vi "SetAnalogOutUI.vi"(8 "Error in":errorcluster, 11 "DevicesAndSignals":T1) -> (0 "Error out":errorcluster, 3 "DevicesAndSignals":T1)   [LabVIEW 2016]
doc: "Use this VI to set selected analog out signals to a certain value."
panel:
  in  "?":dbl(slide) min=-10.0 max=10.0 step=0.01 scale=-10.0..10.0 scale format="%.1g"
  in  "SetAnalogOut":bool
  in  "Signals":i32(listbox)
  in  "stop":bool caption="Stopp"
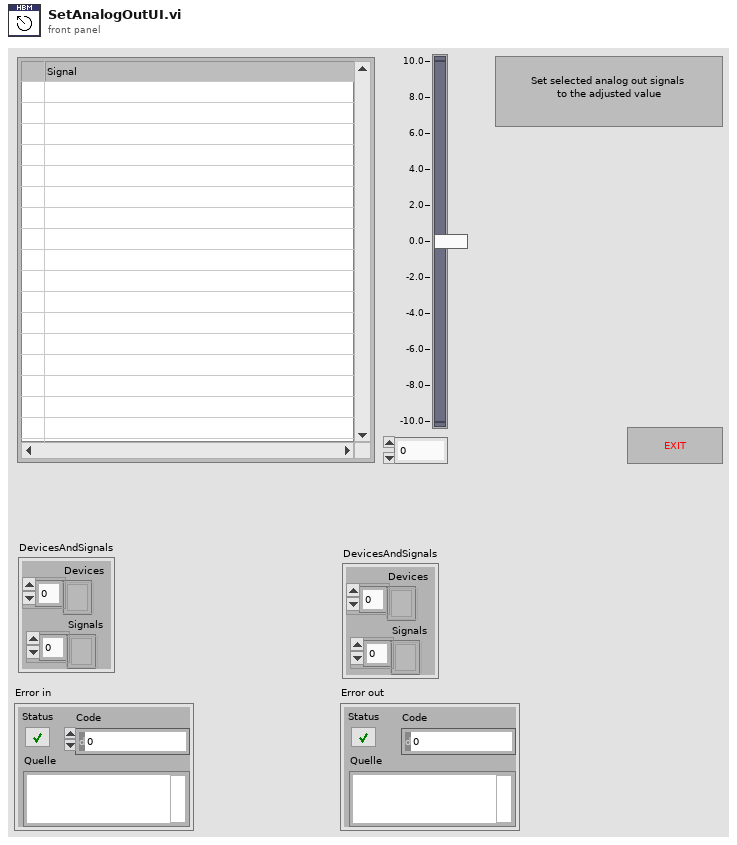
[diagram p1: front panel]
types:
  T1 = cluster{"Devices":refnum<k24>[], "Signals":refnum<k24>[]}
  T2 = typedef "LVPoint32TypeDef.ctl" = cluster{"Horizontal":i32, "Vertical":i32}
  T3 = typedef "LVRowAndColumnTypeDef.ctl" = cluster{"Row":i32, "Column":i32}
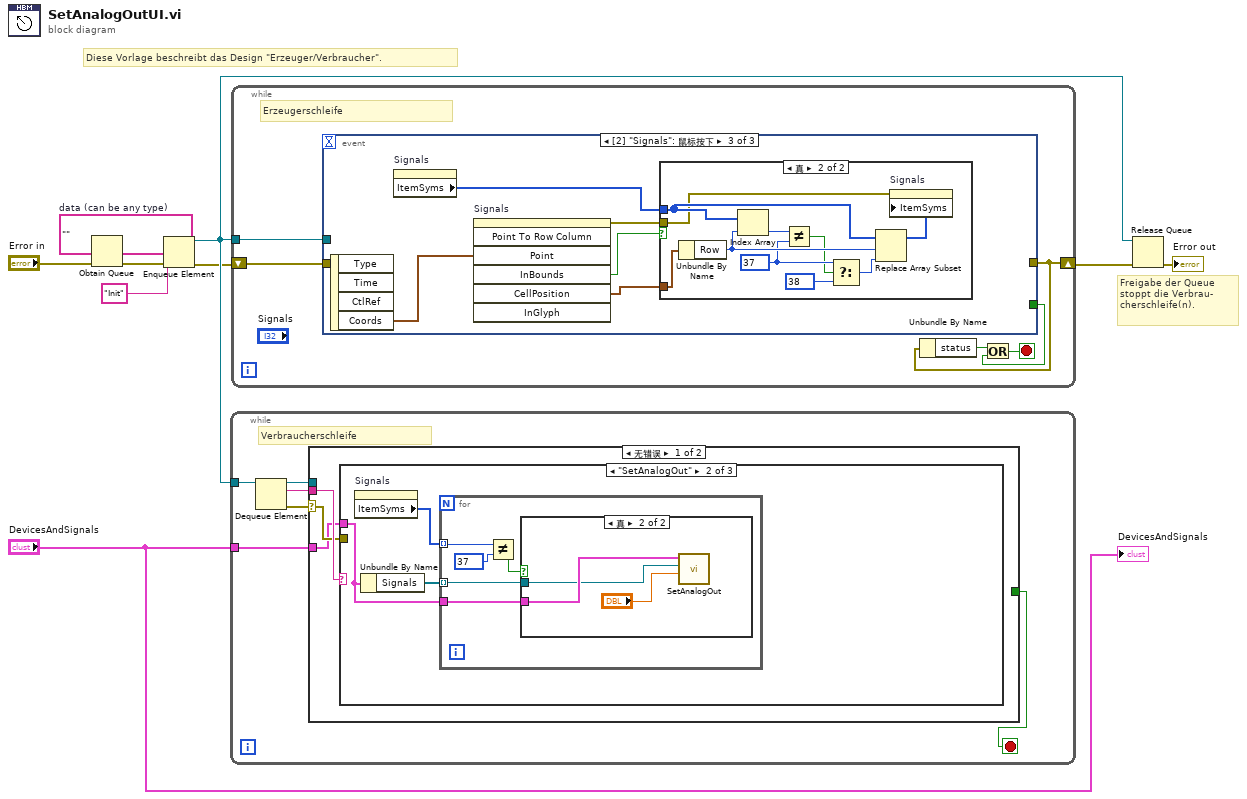
[diagram p0: block diagram]
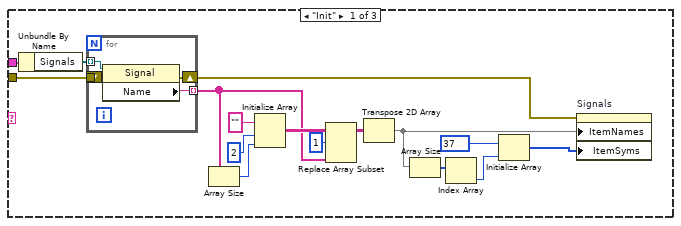
[diagram p2: hidden frame]
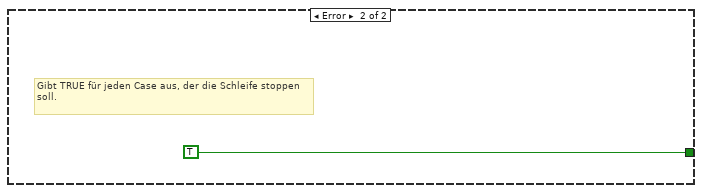
[diagram p5: hidden frame]
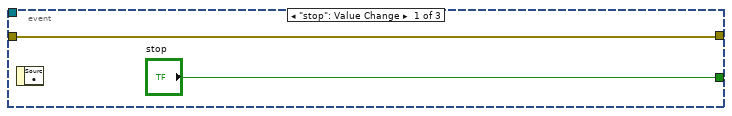
[diagram p6: hidden frame]
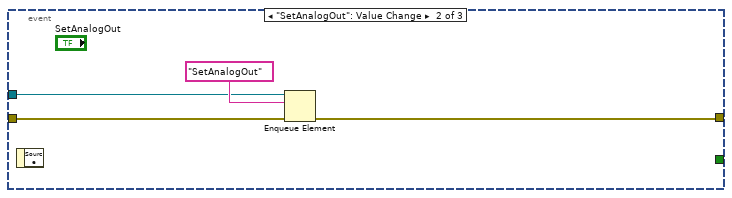
[diagram p7: hidden frame]
diagram:
  w9 = ""  # data (can be any type)
  # "Freigabe der Queue stoppt die Verbrau-\ncherschleife(n)."
  # "Diese Vorlage beschreibt das Design \"Erzeuger/Verbraucher\"."
  n1 = Obtain Queue(element data type=w9, error in (no error)="Error in") -> (queue out=w8:refnum<queue>, error out=w7:errorcluster)  [unwired: 3 in, 1 out]
  n2 = Enqueue Element(queue=w8, element="Init" ("Element"), error in (no error)=w7) -> (queue out=w6:refnum<queue>, error out=w5:errorcluster)  [unwired: 1 in, 1 out]
  n3 = while {
    tunnel: w6 -> [w16]
    tunnel: "DevicesAndSignals" -> [w12]
    stop <- w11 stop-if-true
    # "Verbraucherschleife"
    n4 = Dequeue Element(queue=w16) -> (queue out=w14:refnum<queue>, element=w15:string, error out=w13:errorcluster)  [unwired: 2 in, 1 out]
    n5 = case shown="无错误" w13 {
      selector: w13 -> [w18 _]
      tunnel: w15 -> [w19 _]
      tunnel: [_ TRUE] -> w11
      tunnel: w14 -> [_ _]
      tunnel: w12 -> [w17 _]
      frame No Error {
        n6 = case shown="\"SetAnalogOut\"" w19 {
          tunnel: w18 -> [w24 _ _]
          tunnel: w17 -> [w23 w40 _]
          frame "Init" {
            n7 = Unbundle By Name(w23) -> ("Signals"=w35:refnum<k24>[])
            n8 = for {
              tunnel: [w39] -> w25 mode=indexing
              tunnel: w24 -> [w38]
              tunnel: w35 -> [w37] mode=indexing
              shift-right: [w36] -> w22
              shift-left: _ -> [_]
              n9 = property on="Eigenschaftsknoten" class="Signal"(reference=w37, error in=w38) -> (error out=w36:errorcluster, "Name"=w39:string)  [unwired: 1 out]
            }
            n10 = Array Size(array=w25) -> (size(s)=w29:i32)
            n11 = Initialize Array("" ("Element"), 2 ("Dimension"), w29) -> (w33:string[][])
            n12 = Replace Array Subset(array=w33, new element=w25, index (row)=1 ("Index (Zeile)")) -> (w31:string[][])  [unwired: 1 in]
            n13 = Transpose 2D Array(2D array=w31) -> (transposed array=w21:string[][])
            n14 = Array Size(array=w21) -> (size(s)=w28:i32[])
            n15 = Index Array(array=w28) -> (element=w27:i32)  [unwired: 1 in]
            n16 = Initialize Array(37, w27) -> (w20:i32[])
            n17 = property on="Signals" class="MCListbox (严格)"(error in=w22, "ItemNames"=w21, "ItemSyms"=w20) -> ()  [unwired: 1 in, 2 out]
          }
          frame "SetAnalogOut" {
            n18 = property on="Signals" class="MCListbox (严格)"() -> ("ItemSyms"=w42:i32[])  [unwired: 2 in, 2 out]
            n19 = Unbundle By Name(w40) -> ("Signals"=w41:refnum<k24>[])
            n20 = for {
              tunnel: w42 -> [w46] mode=indexing
              tunnel: w41 -> [w43] mode=indexing
              tunnel: w40 -> [w44]
              n21 = Not Equal?(x=w46, y=37) -> (x != y?=w45:bool)
              n22 = case shown="真" w45 {
                tunnel: w44 -> [_ w50]
                tunnel: w43 -> [_ w49]
                frame False {
                }
                frame True {
                  n23 = call "SetAnalogOut.vi"("Value"="?", "Signal"=w49, "DevicesAndSignals"=w50) -> ()  [unwired: 7 in, 2 out]
                }
              }
            }
          }
          frame Default {
          }
        }
      }
      frame Error {
        # "Gibt TRUE für jeden Case aus, der die Schleife stoppen soll."
      }
    }
  }
  n24 = while {
    shift-right: [w53] -> w10
    shift-left: w5 -> [w56]
    tunnel: w6 -> [w57]
    stop <- w54 stop-if-true
    # "Erzeugerschleife"
    n25 = event shown="[2] \"Signals\": 鼠标按下" {
      selector: _ -> [_ _ _]
      dyn-events: _ -> [_ _ _]
      timeout: _ -> [_ _ _]
      tunnel: w57 -> [_ w62 _]
      tunnel: w56 -> [w58 w61 _]
      tunnel: [w58 w60 _] -> w53
      tunnel: ["stop" _ _] -> w55
      event "stop": Value Change {
        n26 = event-data() -> ()  [unwired: 1 in, 1 out]
      }
      event "SetAnalogOut": Value Change {
        n27 = event-data() -> ()  [unwired: 1 in, 1 out]
        n28 = Enqueue Element(queue=w62, element="SetAnalogOut", error in (no error)=w61) -> (error out=w60:errorcluster)  [unwired: 1 in, 2 out]
      }
      event "Signals": Mouse Down {
        n29 = event-data() -> ("Coords"=w65:T2)  [unwired: 1 in, 3 out]
        n30 = property on="Signals" class="MCListbox (严格)"() -> ("ItemSyms"=w67:i32[])  [unwired: 2 in, 2 out]
        n31 = invoke on="Signals" class="MehrSpaltFeld (strikt)" method="Point To Row Column"("Point"=w65) -> (error out=w66:errorcluster, "InBounds"=w64:bool, "CellPosition"=w68:T3)  [unwired: 6 in, 4 out]
        n32 = case shown="真" w64 {
          tunnel: w68 -> [_ w72]
          tunnel: w67 -> [_ w71]
          tunnel: w66 -> [_ w69]
          frame False {
          }
          frame True {
            w74 = 37
            n33 = Unbundle By Name(w72) -> ("Row"=w78:i32)
            n34 = Index Array(array=w71, index=w78) -> (element=w75:i32)
            n35 = Not Equal?(x=w75, y=w74) -> (x != y?=w73:bool)
            n36 = Select(t=w74, s=w73, f=38) -> (s? t:f=w76:i32)
            n37 = Replace Array Subset(array=w71, new element=w76, index=w78) -> (w70:i32[])
            n38 = property on="Signals" class="MCListbox (严格)"(error in=w69, "ItemSyms"=w70) -> ()  [unwired: 1 in, 2 out]
          }
        }
      }
    }
    n39 = Unbundle By Name(w53) -> ("status"=w52:bool)
    n40 = Or(x=w52, y=w55) -> (x .or. y?=w54:bool)
  }
  n41 = Release Queue(queue=w6, error in (no error)=w10) -> (error out=→"Error out":errorcluster)  [unwired: 1 in, 2 out]
  "DevicesAndSignals" <- "DevicesAndSignals"
